vi "file_sync_v.vi"() -> ()   [LabVIEW 2010]
panel:
  in  "Refresh":bool
  in  "overwrite":bool caption="overwrite?"
  in  "stop":bool
  in  "right2left":bool
  in  "left2right":bool
  in  "right":path
  out "right_t":string[][](table)
  out "left_t":string[][](table)
  in  "left":path
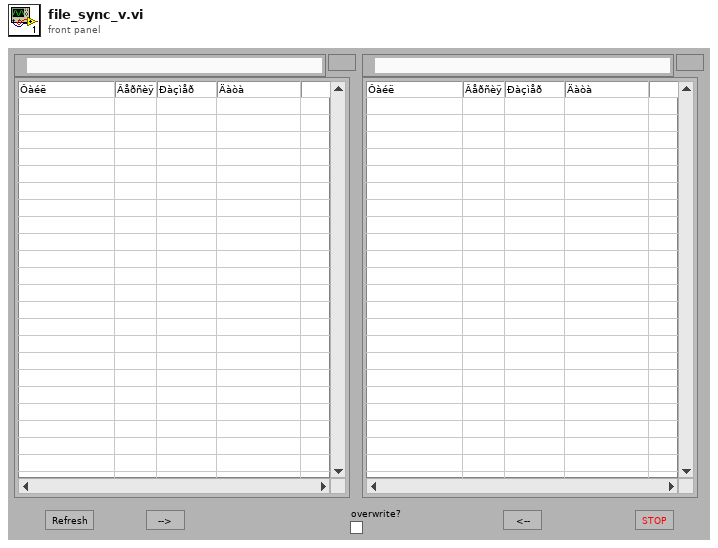
[diagram p1: front panel]
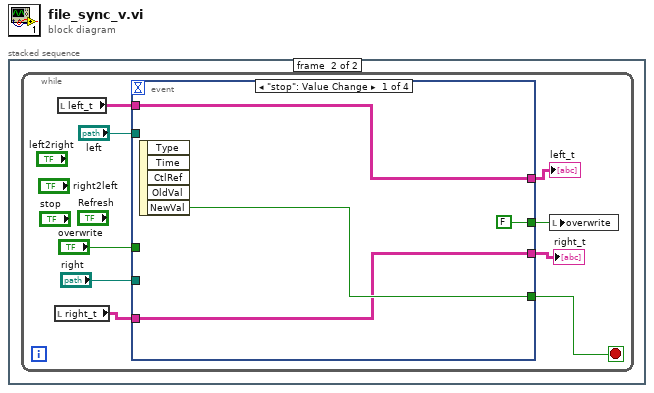
[diagram p0: block diagram]
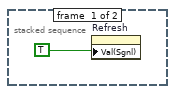
[diagram p2: hidden frame]
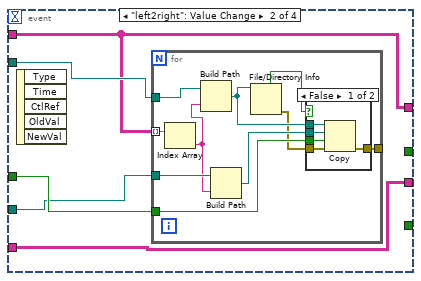
[diagram p3: hidden frame]
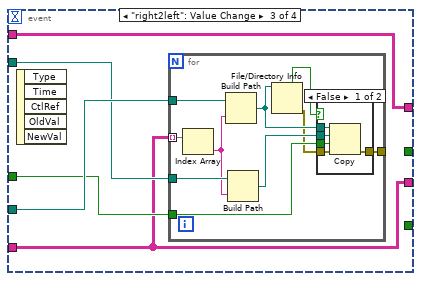
[diagram p5: hidden frame]
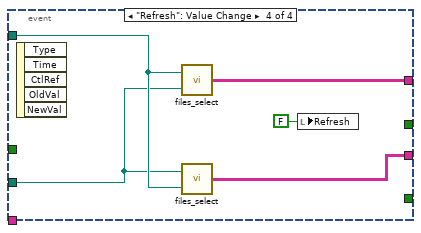
[diagram p7: hidden frame]
diagram:
  n1 = stacked-sequence {
    frame #0 {
      n2 = property on="Refresh" class="Bool (strict)"("Val(Sgnl)"=TRUE) -> ()  [unwired: 2 in, 2 out]
    }
    frame #1 {
      n3 = while {
        stop <- w10 stop-if-true
        n4 = local read "right_t"() -> (w3:string[][])
        n5 = local read "left_t"() -> (w4:string[][])
        n6 = event shown="[0] \"stop\": Value Change" {
          selector: _ -> [_ _ _ _]
          dyn-events: _ -> [_ _ _ _]
          timeout: _ -> [_ _ _ _]
          tunnel: [w14 _ _ _] -> w10
          tunnel: "overwrite" -> [_ w19 w38 _]
          tunnel: "left" -> [_ w18 w39 w61]
          tunnel: "right" -> [_ w17 w40 w60]
          tunnel: [w13 w16 w36 w58] -> w6
          tunnel: [w12 w15 w37 w57] -> w5
          tunnel: w4 -> [w13 w16 w36 _]
          tunnel: w3 -> [w12 w15 w37 _]
          tunnel: [FALSE _ _ _] -> w2
          event "stop": Value Change {
            n7 = event-data() -> ("NewVal"=w14:bool)  [unwired: 1 in, 4 out]
          }
          event "left2right": Value Change {
            n8 = event-data() -> ()  [unwired: 1 in, 5 out]
            n9 = for {
              tunnel: w18 -> [w29]
              tunnel: w16 -> [w28] mode=indexing
              tunnel: w17 -> [w27]
              tunnel: [w24] -> _
              tunnel: w19 -> [w23]
              n10 = Index Array(array=w28) -> (element=w26:string)  [unwired: 1 in]
              n11 = Build Path(base path=w29, name or relative path=w26) -> (appended path=w22:path)
              n12 = Build Path(base path=w27, name or relative path=w26) -> (appended path=w25:path)
              n13 = File/Directory Info(path=w22) -> (directory=w21:bool, error out=w20:errorcluster)  [unwired: 1 in, 5 out]
              n14 = case shown="False" w21 {
                tunnel: w25 -> [w34 _]
                tunnel: [w33 w35] -> w24
                tunnel: w23 -> [w32 _]
                tunnel: w22 -> [w31 _]
                tunnel: w20 -> [w30 w35]
                frame False {
                  n15 = Copy(8:w30, 9:w32, 10:w34, 11:w31) -> (0:w33:errorcluster)  [unwired: 1 in, 2 out]
                }
                frame True {
                }
              }
            }
          }
          event "right2left": Value Change {
            n16 = event-data() -> ()  [unwired: 1 in, 5 out]
            n17 = for {
              tunnel: w40 -> [w50]
              tunnel: w37 -> [w49] mode=indexing
              tunnel: w39 -> [w48]
              tunnel: [w45] -> _
              tunnel: w38 -> [w44]
              n18 = Index Array(array=w49) -> (element=w47:string)  [unwired: 1 in]
              n19 = Build Path(base path=w50, name or relative path=w47) -> (appended path=w43:path)
              n20 = Build Path(base path=w48, name or relative path=w47) -> (appended path=w46:path)
              n21 = File/Directory Info(path=w43) -> (directory=w41:bool, error out=w42:errorcluster)  [unwired: 1 in, 5 out]
              n22 = case shown="False" w41 {
                tunnel: w43 -> [w55 _]
                tunnel: w46 -> [w54 _]
                tunnel: [w53 w56] -> w45
                tunnel: w44 -> [w52 _]
                tunnel: w42 -> [w51 w56]
                frame False {
                  n23 = Copy(8:w51, 9:w52, 10:w54, 11:w55) -> (0:w53:errorcluster)  [unwired: 1 in, 2 out]
                }
                frame True {
                }
              }
            }
          }
          event "Refresh": Value Change {
            n24 = event-data() -> ()  [unwired: 1 in, 5 out]
            n25 = call "files_select.vi"("right"=w60, "left"=w61) -> ("Array"=w58:string[][])
            n26 = call "files_select.vi"("right"=w61, "left"=w60) -> ("Array"=w57:string[][])
            n27 = local write "Refresh"(FALSE ("Refresh")) -> ()
          }
        }
        "left_t" <- w6
        "right_t" <- w5
        n28 = local write "overwrite"(w2) -> ()
      }
    }
  }
